vi "Scan Engine EtherCAT Master.vi"(8 "error in (no error)":errorcluster, 11 "Node Ptr":T1 format="%.0x") -> (0 "error out":errorcluster)   [LabVIEW 2020, in "SEECD System Explorer.lvlib"]
uses:
  SEECD System Explorer.lvlib
  <vilib>/NI VeriStand/Custom Device API/Custom Device API.lvlib
  Shared/Globals/Property Strings.vi
  Shared/SEECD Shared.lvlib
  <vilib>/NI VeriStand/Custom Device API/Get Item Property (U32).vi
  <vilib>/NI VeriStand/Custom Device API/Set Item Property (U32).vi
  Shared/Globals/RT Globals.vi
  <vilib>/NI VeriStand/Custom Device API/Custom Device Item Ref.ctl
panel:
  in  "SHDocVw.IWebBrowser2":refnum<k7>(container)
  in  "Cyclic Data Bandwidth (%)":u32=40 max=100
  in  "Add EtherCAT Slave":bool
  in  "Master ID":u32
  in  "Header":cluster{"Section Name":string}={"Section Name"="EtherCAT Master Settings"}
  in  "Name":string
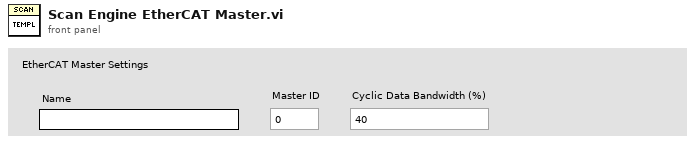
[diagram p1: front panel]
types:
  T1 = typedef "Custom Device API.lvlib/Custom Device Item Ref.ctl" = u64
  T2 = typedef "Custom Device API.lvlib/Custom Device Commands.ctl" = enum16{"Default", "Item renamed", "Shutdown", "Dynamic button pressed"}
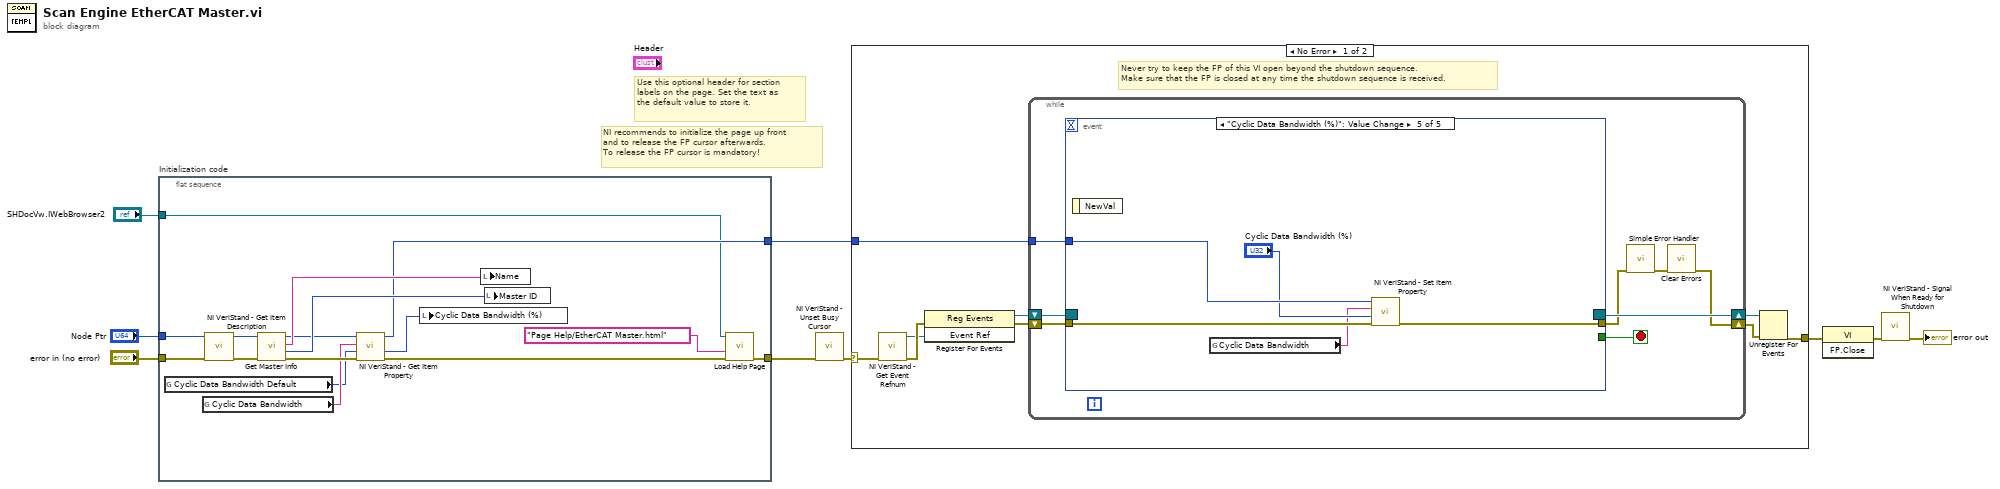
[diagram p0: block diagram]
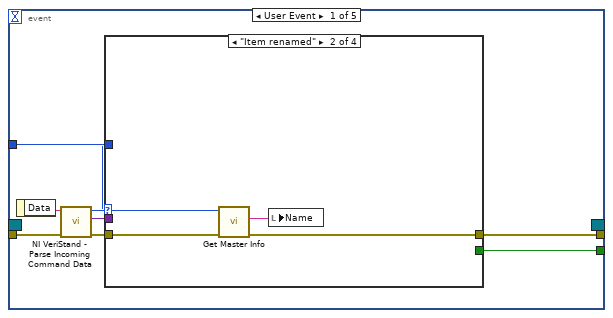
[diagram p2: hidden frame]
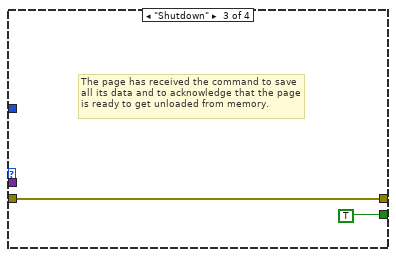
[diagram p4: hidden frame]
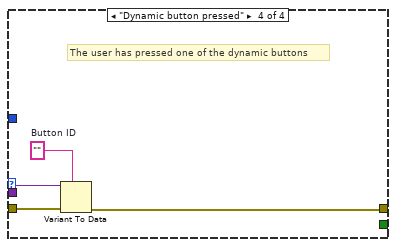
[diagram p5: hidden frame]
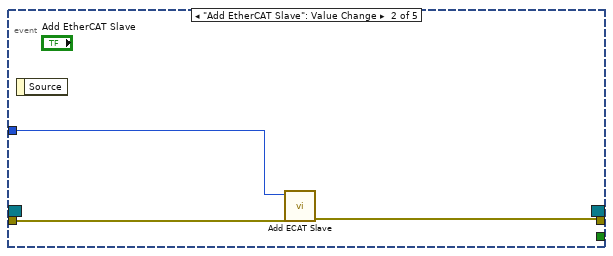
[diagram p6: hidden frame]
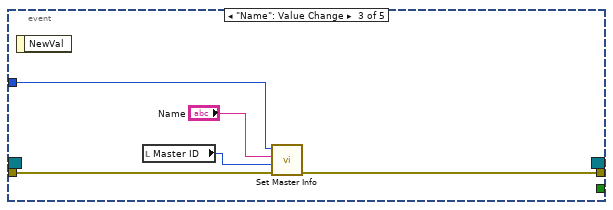
[diagram p7: hidden frame]
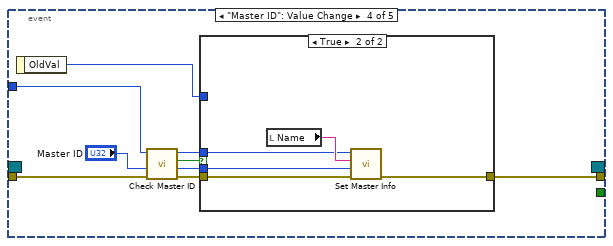
[diagram p8: hidden frame]
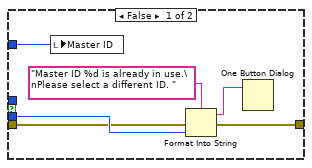
[diagram p9: hidden frame]
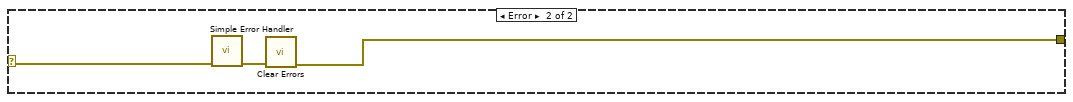
[diagram p10: hidden frame]
diagram:
  # "Use this optional header for section labels on the page. Set the text as the default value to store it."
  # "NI recommends to initialize the page up front\nand to release the FP cursor afterwards.\nTo release the FP cursor is mandatory!"
  n1 = flat-sequence "Initialization code" {
    tunnel: "error in (no error)" -> [w25]
    tunnel: "Node Ptr" -> [w24]
    tunnel: [w15] -> w3
    tunnel: "SHDocVw.IWebBrowser2" -> [w10]
    tunnel: [w11] -> w1
    frame #0 {
      n2 = global read "RT Globals.vi" "Cyclic Data Bandwidth Default"() -> (w14:u32)
      n3 = global read "Property Strings.vi" "Cyclic Data Bandwidth"() -> (w17:string)
      n4 = call <vilib>:"NI VeriStand - Get Item Description.vi"("error in (no error)"=w25, "Item Ref in"=w24) -> ("error out"=w22:errorcluster, "Item Ref out"=w23:T1)  [unwired: 8 out]
      n5 = call "Get Master Info.vi"("error in (no error)"=w22, "Item Ref in"=w23) -> ("error out"=w18:errorcluster, "Master #"=w20:u32, "Master Name"=w21:string, "Item Ref out"=w19:T1)  [unwired: 6 in]
      n6 = call-poly <vilib>:"NI VeriStand - Get Item Property.vi"("error in (no error)"=w18, "Default Value"=w14, "Property Name"=w17, "Item Ref in"=w19) -> ("error out"=w12:errorcluster, "Value"=w16:u32, "Item Ref out"=w15:T1)  [unwired: 4 in, 1 out]
      n7 = local write "Cyclic Data Bandwidth (%)"(w16) -> ()
      n8 = local write "Name"(w21) -> ()
      n9 = local write "Master ID"(w20) -> ()
      n10 = call "Load Help Page.vi"("error in (no error)"=w12, "HTML File to Load"="Page Help/EtherCAT Master.html" ("name or relative path"), "Browser"=w10) -> ("error out"=w11:errorcluster)  [unwired: 8 in]
    }
  }
  n11 = call <vilib>:"NI VeriStand - Unset Busy Cursor.vi"("error in (no error)"=w1) -> ("error out"=w5:errorcluster)  [unwired: 10 out]
  n12 = case shown="No Error" w5 {
    selector: w5 -> [w26 w97]
    tunnel: [w31 w95] -> w9
    tunnel: w3 -> [w27 _]
    frame No Error {
      # "Never try to keep the FP of this VI open beyond the shutdown sequence.\nMake sure that the FP is closed at any time the shutdown sequence is received."
      n13 = call <vilib>:"NI VeriStand - Get Event Refnum.vi"("error in (no error)"=w26) -> ("error out"=w34:errorcluster, "Event Ref"=w30:refnum<user-event>)  [unwired: 9 out]
      n14 = register-events(error in=w34, w30) -> (reference out=w28:refnum<event-registration>, error out=w29:errorcluster)  [unwired: 1 in]
      n15 = while {
        tunnel: w27 -> [w38]
        shift-right: [w35] -> w32
        shift-left: w29 -> [w41]
        shift-right: [w42] -> w33
        shift-left: w28 -> [w40]
        stop <- w39 stop-if-true
        n16 = event shown="[4] \"Cyclic Data Bandwidth (%)\": Value Change" {
          selector: w40 -> [_ _ _ _ _]
          dyn-events: [_ _ _ _ _] -> w42
          timeout: _ -> [_ _ _ _ _]
          tunnel: w41 -> [w50 w64 w69 w77 w94]
          tunnel: [w46 _ _ _ _] -> w39
          tunnel: [w45 w62 w68 w78 w90] -> w37
          tunnel: w38 -> [w44 w63 w66 w75 w93]
          event User Event {
            n17 = event-data() -> ("Data"=w49:string)  [unwired: 1 out]
            n18 = call <vilib>:"NI VeriStand - Parse Incoming Command Data.vi"("error in (no error)"=w50, "Incoming data"=w49) -> ("error out"=w48:errorcluster, "Outgoing data"=w43:variant, "Action"=w47:T2)  [unwired: 7 out]
            n19 = case shown="\"Item renamed\"" w47 {
              tunnel: w48 -> [w51 w54 w56 w61]
              tunnel: [_ _ TRUE _] -> w46
              tunnel: [w51 w52 w56 w58] -> w45
              tunnel: w44 -> [_ w55 _ _]
              tunnel: w43 -> [_ _ _ w60]
              frame "Default", Default {
              }
              frame "Item renamed" {
                n20 = call "Get Master Info.vi"("error in (no error)"=w54, "Item Ref in"=w55) -> ("error out"=w52:errorcluster, "Master Name"=w53:string)  [unwired: 6 in, 2 out]
                n21 = local write "Name"(w53) -> ()
              }
              frame "Shutdown" {
                # "The page has received the command to save all its data and to acknowledge that the page is ready to get unloaded from memory."
              }
              frame "Dynamic button pressed" {
                w59 = ""  # Button ID
                # "The user has pressed one of the dynamic buttons"
                n22 = Variant To Data(error in=w61, type=w59, Variant=w60) -> (error out=w58:errorcluster)  [unwired: 1 out]
              }
            }
          }
          event "Add EtherCAT Slave": Value Change {
            n23 = event-data() -> ()  [unwired: 2 out]
            n24 = call "Add ECAT Slave.vi"("error in (no error)"=w64, "ECAT Master Ref in"=w63) -> ("error out"=w62:errorcluster)  [unwired: 8 in, 1 out]
          }
          event "Name": Value Change {
            n25 = event-data() -> ()  [unwired: 2 out]
            n26 = local read "Master ID"() -> (w65:u32)
            n27 = call "Set Master Info.vi"("error in (no error)"=w69, "Master #"=w65, "Master Name"="Name", "Item Ref in"=w66) -> ("error out"=w68:errorcluster)  [unwired: 6 in, 1 out]
          }
          event "Master ID": Value Change {
            n28 = event-data() -> ("OldVal"=w70:u32)  [unwired: 1 out]
            n29 = call "Check Master ID.vi"("error in (no error)"=w77, "Master ID in"="Master ID", "Item Ref in"=w75) -> ("error out"=w76:errorcluster, "Master ID out"=w72:u32, "Available?"=w71:bool, "Item Ref out"=w74:T1)  [unwired: 5 in]
            n30 = case shown="True" w71 {
              tunnel: [w80 w89] -> w78
              tunnel: w76 -> [w81 w87]
              tunnel: w74 -> [_ w86]
              tunnel: w72 -> [w83 w85]
              tunnel: w70 -> [w79 _]
              frame False {
                n31 = local write "Master ID"(w79) -> ()
                n32 = Format Into String(format string="Master ID %d is already in use.\nPlease select a different ID. ", error in=w81, w83) -> (resulting string=w82:string, error out=w80:errorcluster)  [unwired: 1 in]
                n33 = One Button Dialog(message=w82) -> ()  [unwired: 1 in, 1 out]
              }
              frame True {
                n34 = local read "Name"() -> (w88:string)
                n35 = call "Set Master Info.vi"("error in (no error)"=w87, "Master #"=w85, "Master Name"=w88, "Item Ref in"=w86) -> ("error out"=w89:errorcluster)  [unwired: 6 in, 1 out]
              }
            }
          }
          event "Cyclic Data Bandwidth (%)": Value Change {
            n36 = event-data() -> ()  [unwired: 2 out]
            n37 = global read "Property Strings.vi" "Cyclic Data Bandwidth"() -> (w91:string)
            n38 = call-poly <vilib>:"NI VeriStand - Set Item Property.vi"("error in (no error)"=w94, "Value"="Cyclic Data Bandwidth (%)", "Property Name"=w91, "Item Ref in"=w93) -> ("error out"=w90:errorcluster)  [unwired: 5 in, 2 out]
          }
        }
        n39 = call <vilib>:"Simple Error Handler.vi"("error in (no error)"=w37) -> ("error out"=w36:errorcluster)  [unwired: 1 in, 7 out]
        n40 = call <vilib>:"Clear Errors.vi"("error in (no error)"=w36) -> ("error out"=w35:errorcluster)  [unwired: 1 in, 5 out]
      }
      n41 = Unregister For Events(event registration refnum=w33, error in=w32) -> (error out=w31:errorcluster)
    }
    frame Error {
      n42 = call <vilib>:"Simple Error Handler.vi"("error in (no error)"=w97) -> ("error out"=w96:errorcluster)  [unwired: 1 in, 7 out]
      n43 = call <vilib>:"Clear Errors.vi"("error in (no error)"=w96) -> ("error out"=w95:errorcluster)  [unwired: 1 in, 5 out]
    }
  }
  n44 = invoke class="VI" method="FP.Close"(error in=w9) -> (error out=w8:errorcluster)  [unwired: 2 in, 2 out]
  n45 = call <vilib>:"NI VeriStand - Signal When Ready for Shutdown.vi"("error in (no error)"=w8) -> ("error out"=→"error out":errorcluster)  [unwired: 10 out]
